vi "Main.vi"(11 "Module Admin":refnum<class "Delacor_lib_QMH_Cloneable Module Admin.lvclass">) -> ()   [LabVIEW 2020, in "TCP Client.lvlib"]
doc: "This template is based off of the Queued Message Handler design pattern and the Queued Message Handler project template that ships with LabVIEW.\n\nThe main difference is that the queue is private to this module and communication between modules is performed via Broadcast and Request events.\n\nRequest events are wrapped in public API methods and are handled in the Event Handling Loop (EHL) of this VI. Any module can register for Broadcast events sent by this module. The EHL generates messages based on user interface actions.\n\nThe Message Handling Loop (MHL) processes messages generated by the EHL, or by other messages. The messages are string values, so new messages can be added easily to the Message Cases case structure in the MHL. Each message cluster can also provide an optional value for Message Data, which is a variant that can be converted to whatever message-specific data is required.\n_____\nBased on Delacor QMH Project Template 6.0.0.89."
uses:
  TCP Client.lvlib
  <vilib>/Delacor/Delacor QMH/Libraries/Cloneable Module Admin_class/Delacor_lib_QMH_Cloneable Module Admin.lvclass
  C:/Program Files (x86)/National Instruments/LabVIEW 2020/vi.lib/Delacor/Delacor QMH/Libraries/Module Admin_class/Delacor_lib_QMH_Module Admin.lvclass
  Module Data--cluster.ctl
  <vilib>/Delacor/Delacor QMH/Libraries/Message Queue_class/Delacor_lib_QMH_Message Queue.lvclass/Delacor_lib_QMH_Message Queue.ctl
  <vilib>/Delacor/Delacor QMH/Libraries/Cloneable Module Admin_class/Delacor_lib_QMH_Cloneable Module Admin.lvclass/Delacor_lib_QMH_Cloneable Module Admin.ctl
  Stop Argument--cluster.ctl
  <vilib>/Delacor/Delacor QMH/Libraries/Module Admin_class/Delacor_lib_QMH_Module Admin.lvclass/Delacor_lib_QMH_Module Admin.ctl
  <vilib>/Utility/miscctls.llb/LVPointTypeDef.ctl
  <vilib>/Delacor/Delacor QMH/Libraries/Message Queue_class/Delacor_lib_QMH_Enqueue Message (Single).vi
  <vilib>/Delacor/Delacor QMH/Libraries/Cloneable Module Admin_class/Delacor_lib_QMH_Get Module ID.vi
  <vilib>/Delacor/Delacor QMH/Libraries/Module Admin_class/Delacor_lib_QMH_Get External Launch.vi
  <vilib>/Utility/error.llb/Error Cluster From Error Code.vi
  <vilib>/ErrorRing/Error Ring.xnode
  <vilib>/Delacor/Delacor QMH/Libraries/Message Queue_class/Delacor_lib_QMH_Message Queue.lvclass
panel:
  out "DATA":T1 {"Knob" scale=0.0..10.0; "Horizontal Pointer Slide" scale=0.0..10.0}
  in  "stop":bool
  out "error out":errorcluster
  out "Status":string
  in  "Simulate EHL Error":bool
  in  "Simulate MHL Error":bool
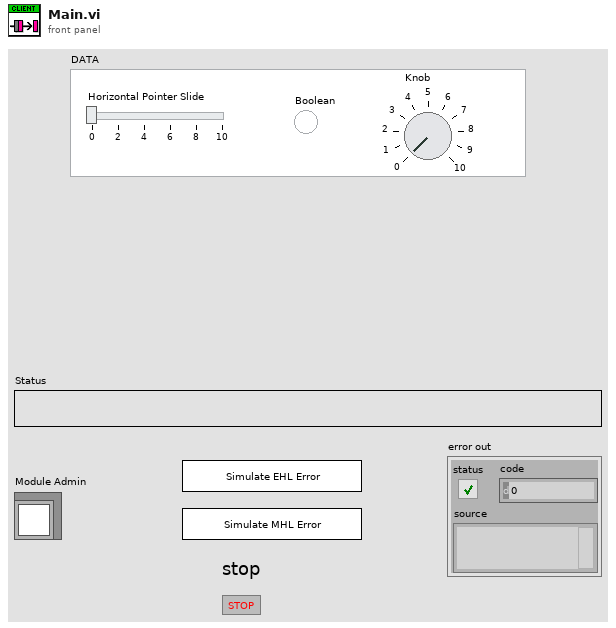
[diagram p1: front panel]
types:
  T1 = cluster{"Horizontal Pointer Slide":dbl, "Boolean":bool, "Knob":dbl}
  T2 = typedef "TCP Client.lvlib/Request Events--cluster.ctl" = cluster{"Stop Module":refnum<user-event>, "Show Panel":refnum<user-event>, "Hide Panel":refnum<user-event>, "Show Diagram":refnum<user-event>, "Get Module Execution Status":refnum<user-event>, "Connect to TCP Server":refnum<user-event>}
  T3 = typedef "TCP Client.lvlib/Module Data--cluster.ctl" = cluster{"Status":string}
  T4 = enum32{"invalid lock state", "Not Locked", "Locked (No Password)", "Password-protected"}
  T5 = typedef "TCP Client.lvlib/Stop Argument--cluster.ctl" = cluster{"Module ID":i32, "Origin":string, "Exit via Stop Module Req?":bool, "Wait for Module to stop?":bool}
  T6 = typedef "LVPointTypeDef.ctl" = cluster{"Horizontal":i16, "Vertical":i16}
  T7 = enum32{"Invalid", "Standard", "Closed", "Hidden", "Minimized", "Maximized"}
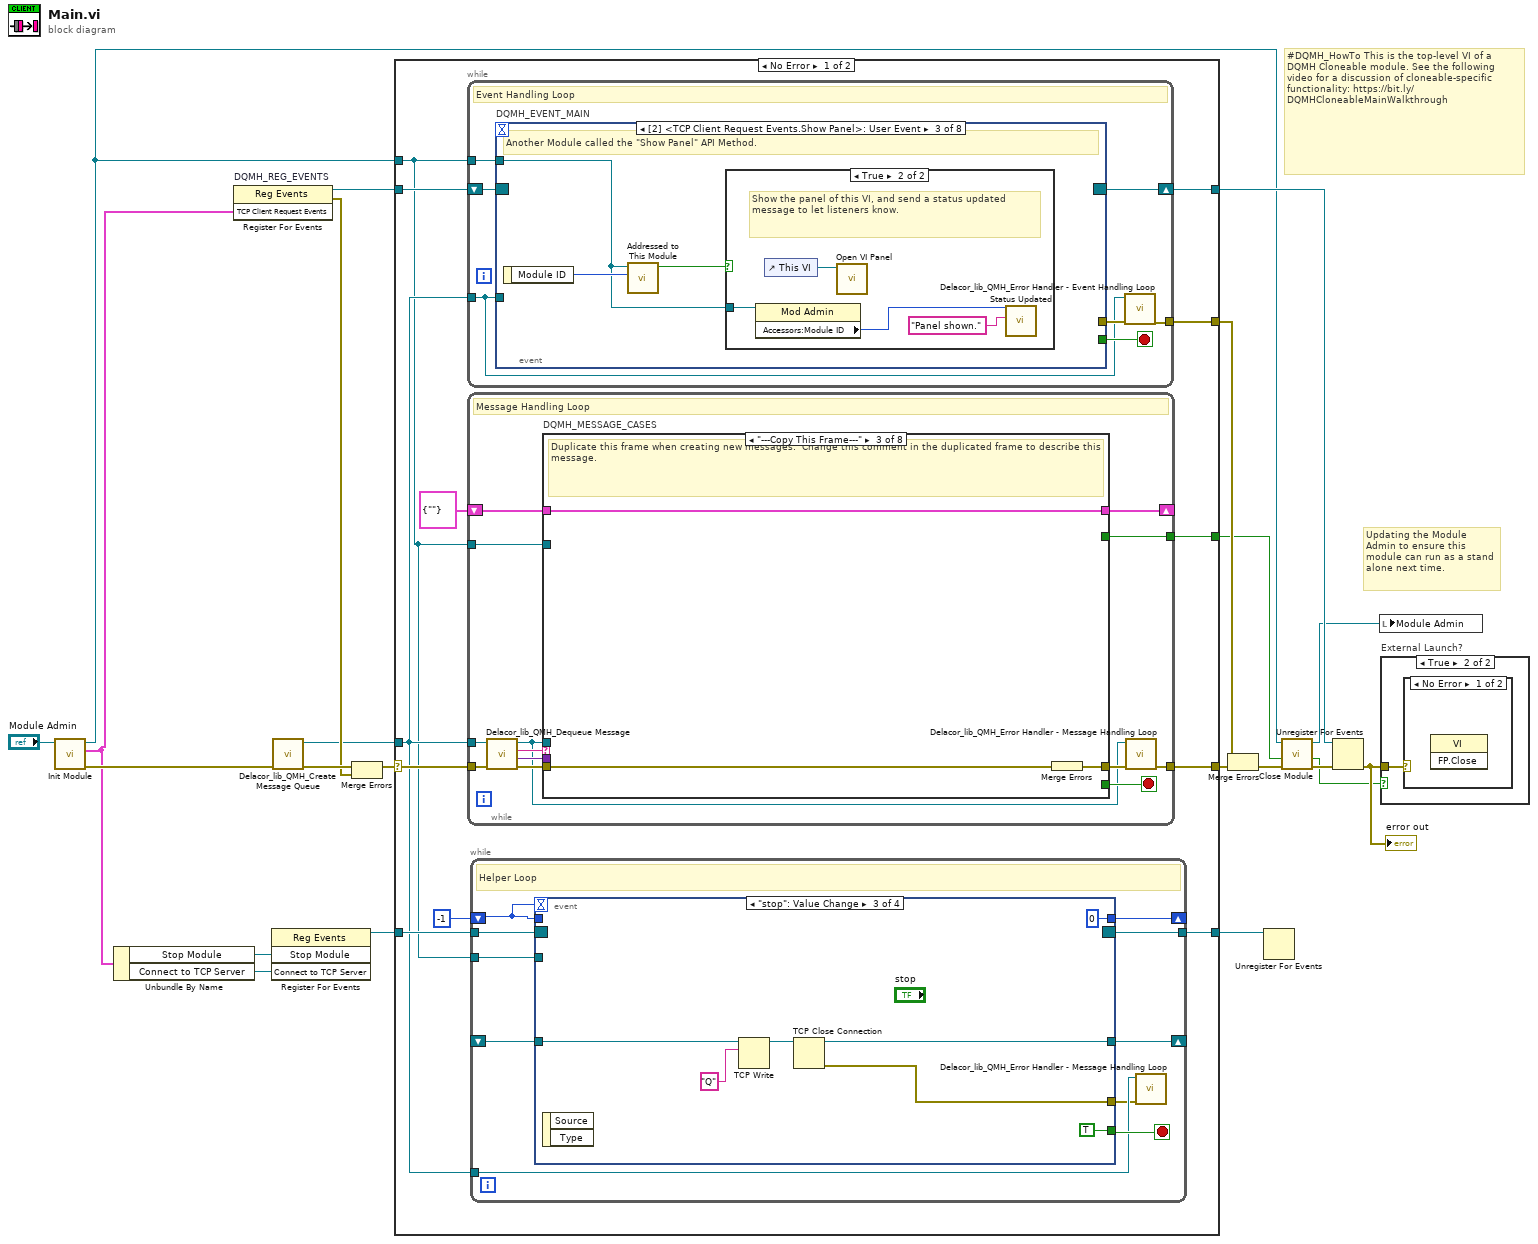
[diagram p0: block diagram]
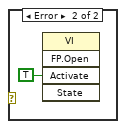
[diagram p3: hidden frame]
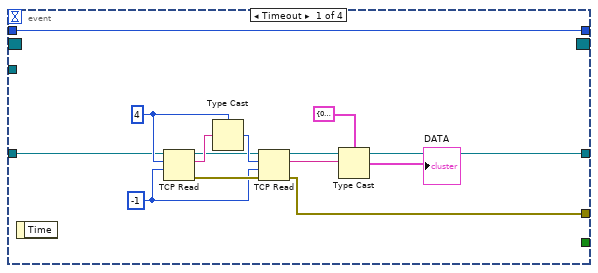
[diagram p4: hidden frame]
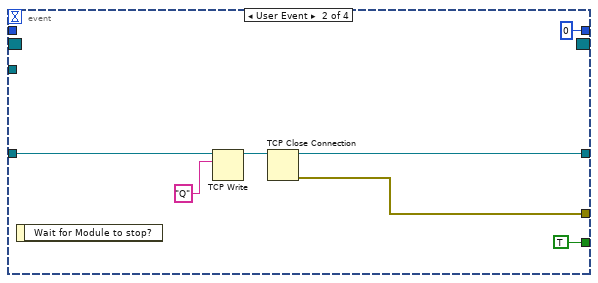
[diagram p5: hidden frame]
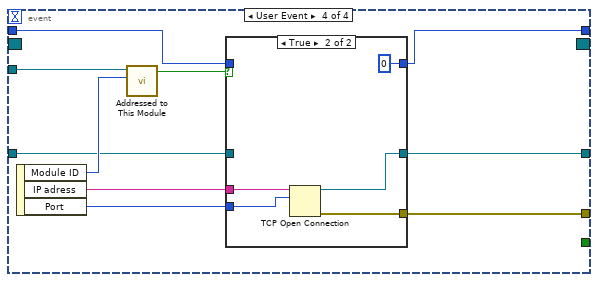
[diagram p6: hidden frame]
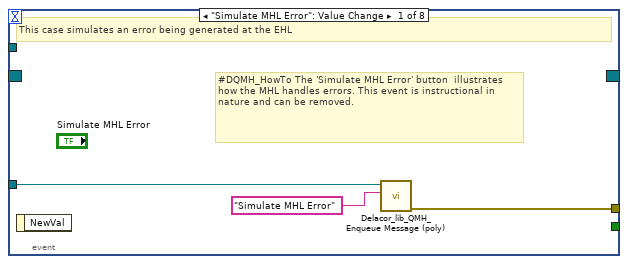
[diagram p8: hidden frame]
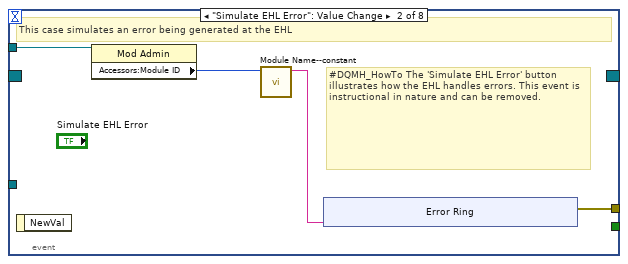
[diagram p9: hidden frame]
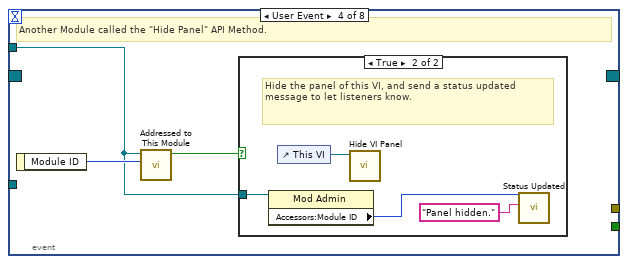
[diagram p11: hidden frame]
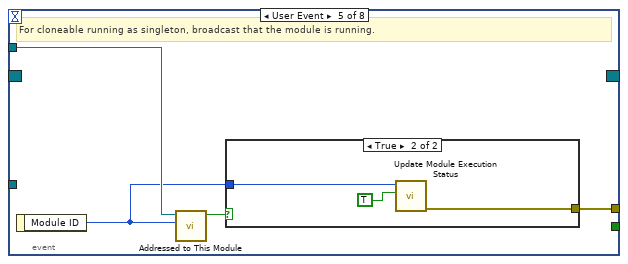
[diagram p13: hidden frame]
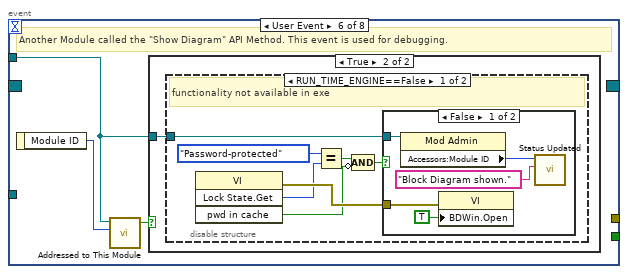
[diagram p15: hidden frame]
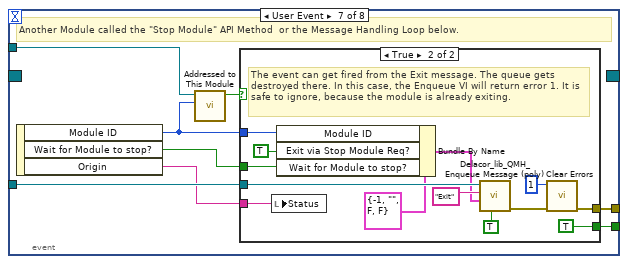
[diagram p19: hidden frame]
diagram:
  # "#DQMH_HowTo This is the top-level VI of a DQMH Cloneable module. See the following video for a discussion of cloneable-specific functionality: https://bit.ly/DQMHCloneableMainWalkthrough"
  # "Updating the Module Admin to ensure this module can run as a stand alone next time."
  n1 = call "Init Module.vi"("Cloneable Module Admin in"="Module Admin") -> ("error out"=w19:errorcluster, "TCP Client Request Events"=w5:T2, "Cloneable Module Admin out"=w9:refnum<class "Delacor_lib_QMH_Cloneable Module Admin.lvclass">)  [unwired: 8 in]
  n2 = Unbundle By Name(w5) -> ("Stop Module"=w4:refnum<user-event>, "Connect to TCP Server"=w1:refnum<user-event>)
  n3 = register-events "DQMH_REG_EVENTS"(w5) -> (reference out=w12:refnum<event-registration>, error out=w14:errorcluster)  [unwired: 2 in]
  n4 = register-events(w4, w1) -> (reference out=w3:refnum<event-registration>)  [unwired: 2 in, 1 out]
  n5 = call <vilib>:"Delacor_lib_QMH_Create Message Queue.vi"("error in"=w19) -> ("error out"=w16:errorcluster, "Message Queue"=w11:refnum<class "Delacor_lib_QMH_Message Queue.lvclass">)  [unwired: 9 in]
  n6 = Merge Errors(w16, w14) -> (w15:errorcluster)
  n7 = case shown="No Error" w15 {
    selector: w15 -> [w32 w285]
    tunnel: [w34 w284] -> w20
    tunnel: [w31 w292] -> w13
    tunnel: w12 -> [w29 w292]
    tunnel: w11 -> [w25 w283]
    tunnel: [w33 _] -> w21
    tunnel: w9 -> [w24 w288]
    tunnel: [w28 _] -> w7
    tunnel: w3 -> [w27 w282]
    tunnel: [w26 w282] -> w2
    frame No Error {
      n8 = while {
        tunnel: w25 -> [w89]
        shift-right: [w92] -> w31
        shift-left: w29 -> [w93]
        tunnel: [w94] -> w33
        tunnel: w24 -> [w90]
        stop <- w91 stop-if-true
        # "Event Handling Loop"
        n9 = event "DQMH_EVENT_MAIN" shown="[2] <TCP Client Request Events.Show Panel>: User Event" {
          selector: w93 -> [_ _ _ _ _ _ _ _]
          dyn-events: [_ _ _ _ _ _ _ _] -> w92
          timeout: _ -> [_ _ _ _ _ _ _ _]
          tunnel: [_ _ _ _ _ _ w150 _] -> w91
          tunnel: w89 -> [w97 _ _ _ _ _ w153 w169]
          tunnel: [w98 w102 _ _ w127 _ w154 w172] -> w95
          tunnel: w90 -> [_ w101 w110 w117 w125 w131 w152 w170]
          event "Simulate MHL Error": Value Change {
            # "#DQMH_HowTo The 'Simulate MHL Error' button  illustrates how the MHL handles errors. This event is instructional in nature and can be removed."
            # "This case simulates an error being generated at the EHL"
            n10 = event-data() -> ()  [unwired: 1 in, 1 out]
            n11 = call-poly <vilib>:"Delacor_lib_QMH_Enqueue Message (poly).vi"("Message"="Simulate MHL Error", "Message Queue in"=w97) -> ("error out"=w98:errorcluster)  [unwired: 8 in, 1 out]
          }
          event "Simulate EHL Error": Value Change {
            # "#DQMH_HowTo The 'Simulate EHL Error' button  illustrates how the EHL handles errors. This event is instructional in nature and can be removed."
            # "This case simulates an error being generated at the EHL"
            n12 = event-data() -> ()  [unwired: 1 in, 1 out]
            n13 = property class="Mod Admin"(reference=w101) -> ("Accessors:Module ID"=w100:i32)  [unwired: 1 in, 2 out]
            n14 = call "Module Name--constant.vi"("Module ID"=w100) -> ("Module Name"=w99:string)  [unwired: 10 in]
            n15 = xnode "Error Ring"("parameter 0"=w99) -> ("error out"=w102:errorcluster)
          }
          event User Event {
            # "Another Module called the \"Show Panel\" API Method."
            n16 = event-data() -> ("Module ID"=w111:i32)  [unwired: 1 in]
            n17 = call "Addressed to This Module.vi"("Module ID from Argument"=w111, "Module Admin"=w110) -> ("Addressed to this instance?"=w112:bool)  [unwired: 8 in, 1 out]
            n18 = case shown="True" w112 {
              tunnel: w110 -> [_ w114]
              frame False {
              }
              frame True {
                # "Show the panel of this VI, and send a status updated message to let listeners know."
                n19 = property class="Mod Admin"(reference=w114) -> ("Accessors:Module ID"=w113:i32)  [unwired: 1 in, 2 out]
                n20 = control-ref of="This VI"() -> (w116:refnum<vi>)
                n21 = call "Open VI Panel.vi"("VI"=w116) -> ()  [unwired: 10 in, 1 out]
                n22 = call "Status Updated.vi"("Status"="Panel shown." ("format string"), "Module ID"=w113) -> ()  [unwired: 9 in, 1 out]
              }
            }
          }
          event User Event {
            # "Another Module called the \"Hide Panel\" API Method."
            n23 = event-data() -> ("Module ID"=w118:i32)  [unwired: 1 in]
            n24 = call "Addressed to This Module.vi"("Module ID from Argument"=w118, "Module Admin"=w117) -> ("Addressed to this instance?"=w119:bool)  [unwired: 8 in, 1 out]
            n25 = case shown="True" w119 {
              tunnel: w117 -> [_ w121]
              frame False {
              }
              frame True {
                # "Hide the panel of this VI, and send a status updated message to let listeners know."
                n26 = property class="Mod Admin"(reference=w121) -> ("Accessors:Module ID"=w120:i32)  [unwired: 1 in, 2 out]
                n27 = control-ref of="This VI"() -> (w123:refnum<vi>)
                n28 = call "Hide VI Panel.vi"("VI"=w123) -> ()  [unwired: 10 in, 1 out]
                n29 = call "Status Updated.vi"("Status"="Panel hidden." ("format string"), "Module ID"=w120) -> ()  [unwired: 9 in, 1 out]
              }
            }
          }
          event User Event {
            # "For cloneable running as singleton, broadcast that the module is running."
            n30 = event-data() -> ("Module ID"=w124:i32)  [unwired: 1 in]
            n31 = call "Addressed to This Module.vi"("Module ID from Argument"=w124, "Module Admin"=w125) -> ("Addressed to this instance?"=w126:bool)  [unwired: 8 in, 1 out]
            n32 = case shown="True" w126 {
              tunnel: [_ w130] -> w127
              tunnel: w124 -> [_ w129]
              frame False {
              }
              frame True {
                n33 = call "Update Module Execution Status.vi"("Running?"=TRUE, "Module ID"=w129) -> ("error out"=w130:errorcluster)  [unwired: 9 in]
              }
            }
          }
          event User Event {
            # "Another Module called the \"Show Diagram\" API Method. This event is used for debugging."
            n34 = event-data() -> ("Module ID"=w132:i32)  [unwired: 1 in]
            n35 = call "Addressed to This Module.vi"("Module ID from Argument"=w132, "Module Admin"=w131) -> ("Addressed to this instance?"=w133:bool)  [unwired: 8 in, 1 out]
            n36 = case shown="True" w133 {
              tunnel: w131 -> [_ w134]
              frame False {
              }
              frame True {
                n37 = disable-structure shown="RUN_TIME_ENGINE==False" {
                  disable-tunnel: w134 -> [w135 _]
                  frame condition #0 (active) {
                    # "functionality not available in exe"
                    n38 = invoke class="VI" method="Lock State.Get"() -> (error out=w141:errorcluster, "Get Lock State"=w140:T4, "pwd in cache"=w137:bool)  [unwired: 4 in, 1 out]
                    n39 = Equal?(x=T4."Password-protected", y=w140) -> (x = y?=w138:bool)
                    n40 = Compound Arithmetic op=AND(w138, invert w137) -> (w136:bool)
                    n41 = case shown="False" w136 {
                      tunnel: w141 -> [w146 _]
                      tunnel: w135 -> [w143 _]
                      frame False {
                        n42 = property class="Mod Admin"(reference=w143) -> ("Accessors:Module ID"=w142:i32)  [unwired: 1 in, 2 out]
                        n43 = property class="VI"(error in=w146, "BDWin.Open"=TRUE ("Block Diagram Window:Open")) -> ()  [unwired: 1 in, 2 out]
                        n44 = call "Status Updated.vi"("Status"="Block Diagram shown." ("format string"), "Module ID"=w142) -> ()  [unwired: 9 in, 1 out]
                      }
                      frame True {
                        # "Password-protected VI, and the password is not in the cache. Do not show the diagram."
                      }
                    }
                  }
                  frame condition #1 {
                  }
                }
              }
            }
          }
          event User Event {
            # "Another Module called the \"Stop Module\" API Method  or the Message Handling Loop below."
            n45 = event-data() -> ("Module ID"=w148:i32, "Wait for Module to stop?"=w149:bool, "Origin"=w147:string)  [unwired: 1 in]
            n46 = call "Addressed to This Module.vi"("Module ID from Argument"=w148, "Module Admin"=w152) -> ("Addressed to this instance?"=w151:bool)  [unwired: 8 in, 1 out]
            n47 = case shown="True" w151 {
              tunnel: [_ w166] -> w154
              tunnel: w153 -> [_ w162]
              tunnel: [_ TRUE] -> w150
              tunnel: w149 -> [_ w157]
              tunnel: w148 -> [_ w159]
              tunnel: w147 -> [_ w155]
              frame False {
              }
              frame True {
                # "The event can get fired from the Exit message. The queue gets destroyed there. In this case, the Enqueue VI will return error 1. It is safe to ignore, because the module is already exiting."
                n48 = local write "Status"(w155) -> ()
                n49 = Bundle By Name(cluster=T5 {"Module ID"=-1, "Origin"="", "Exit via Stop Module Req?"=FALSE, "Wait for Module to stop?"=FALSE} ("Stop Argument"), "Module ID"=w159, "Exit via Stop Module Req?"=TRUE, "Wait for Module to stop?"=w157) -> (w156:T5)
                n50 = call-poly <vilib>:"Delacor_lib_QMH_Enqueue Message (poly).vi"("Priority Message? (F)"=TRUE, "Message Data"=w156, "Message"="Exit", "Message Queue in"=w162) -> ("error out"=w167:errorcluster)  [unwired: 6 in, 1 out]
                n51 = call <vilib>:"Clear Errors.vi"("error in (no error)"=w167, "specific error code to clear (0: all)"=1) -> ("error out"=w166:errorcluster)  [unwired: 4 in, 1 out]
              }
            }
          }
          event Panel Close? {
            w171 = TRUE  # Discard the event, the MHL is responsible for closing and stopping this VI.
            # "Hide the panel or send the 'Exit' message if the user clicks the 'X' on the module main VI panel."
            n52 = event-data() -> ()  [unwired: 1 in, 1 out]
            n53 = property class="Mod Admin"(reference=w170) -> ("Accessors:External Launch"=w168:bool)  [unwired: 1 in, 2 out]
            n54 = case shown="True" w168 {
              tunnel: w169 -> [_ w176]
              tunnel: [_ w177] -> w172
              frame True {
                # "If externally launched, clicking the 'X' hides the panel, but doesn't close it."
                n55 = control-ref of="This VI"() -> (w173:refnum<vi>)
                n56 = call "Hide VI Panel.vi"("VI"=w173) -> ()  [unwired: 10 in, 1 out]
              }
              frame False {
                # "If run as a stand-alone VI, clicking the panel 'X' stops the VI."
                n57 = call-poly <vilib>:"Delacor_lib_QMH_Enqueue Message (poly).vi"("Priority Message? (F)"=TRUE, "Message"="Exit", "Message Queue in"=w176) -> ("error out"=w177:errorcluster)  [unwired: 7 in, 1 out]
              }
            }
            n58 = event-data("Discard?"=w171) -> ()  [unwired: 1 in, 1 out]
          }
        }
        n59 = call-dynamic "Delacor_lib_QMH_Error Handler - Event Handling Loop.vi"("error in"=w95, "Message Queue in"=w89) -> ("dup error in"=w94:errorcluster)  [unwired: 8 in, 1 out]
      }
      n60 = while {
        tunnel: w25 -> [w181]
        shift-right: [w185] -> _
        shift-left: T3 {"Status"=""} ("Data Cluster") -> [w186]
        tunnel: w32 -> [w189]
        tunnel: [w187] -> w34
        tunnel: w24 -> [w179]
        tunnel: [w178] -> w28
        stop <- w184 stop-if-true
        # "Message Handling Loop"
        n61 = call-dynamic "Delacor_lib_QMH_Dequeue Message.vi"("error in"=w189, "Message Queue in"=w181) -> ("error out"=w188:errorcluster, "Message Data"=w182:variant, "Message"=w183:string, "Message Queue out"=w180:refnum<class "Delacor_lib_QMH_Message Queue.lvclass">)  [unwired: 6 in]
        n62 = case "DQMH_MESSAGE_CASES" shown="\"---Copy This Frame---\"" w183 {
          selector: w183 -> [_ _ _ _ _ _ _ w269]
          tunnel: w180 -> [_ _ _ _ w220 _ w259 _]
          tunnel: w188 -> [w209 w213 w216 w218 w229 w242 w265 w271]
          tunnel: [w207 w213 w215 w218 w225 w241 w262 w272] -> w190
          tunnel: w186 -> [w200 w212 w214 w217 w224 w239 w258 w270]
          tunnel: [w199 w212 w214 w217 w224 w239 w258 w270] -> w185
          tunnel: [_ _ _ _ _ _ w257 _] -> w184
          tunnel: w182 -> [_ _ _ _ w223 _ w255 _]
          tunnel: w179 -> [w194 _ _ _ w222 w237 w251 w267]
          tunnel: [_ _ _ _ _ _ w253 _] -> w178
          frame "Initialize" {
            w191 = "Initial Message" ("Initial Message")
            # "#CodeNeeded - Initialize the appearance of the front panel."
            # "#CodeNeeded - Initialize your state data here."
            # "Initialize - Any operation that needs to be done before the module can receive messages. Synchronize Caller Events.vi will inform Start Module.vi that the module has launched and is ready to receive messages. Module Did Init.vi will broadcast that the module initialized."
            n63 = call "Synchronize Caller Events.vi"("error in (no error)"=w209, "Module Admin"=w194) -> ("error out"=w208:errorcluster, "Module Admin out"=w193:refnum<class "Delacor_lib_QMH_Cloneable Module Admin.lvclass">)  [unwired: 8 in]
            n64 = property class="Mod Admin"(reference=w193) -> ("Accessors:Module ID"=w196:i32, "Accessors:External Launch"=w195:bool)  [unwired: 1 in, 2 out]
            n65 = call "Module Name--constant.vi"("Module ID"=w196) -> ("Module Name"=w204:string)  [unwired: 10 in]
            n66 = property class="VI"("Front Panel.Title"=w204) -> (reference out=w206:refnum<vi>, error out=w211:errorcluster)  [unwired: 2 in]
            n67 = Select(t=T7."Hidden" ("State"), s=w195, f=T7."Standard" ("State")) -> (s? t:f=w201:T7)
            n68 = invoke class="VI" method="FP.Open"(reference=w206, error in=w211, "State"=w201) -> (reference out=w205:refnum<vi>, error out=w210:errorcluster)  [unwired: 2 in, 3 out]
            n69 = call "Module Name--constant.vi"("Module ID"=w196) -> ("Module Name"=w197:string)  [unwired: 10 in]
            n70 = Bundle By Name(cluster=w200, "Status"=w191) -> (w199:T3)
            n71 = invoke class="VI" method="FP.Center"(reference=w205, error in=w210) -> ()  [unwired: 1 in, 3 out]
            n72 = property on="Pane" class="Pane"("Origin"=T6 {"Horizontal"=0, "Vertical"=0}) -> ()  [unwired: 2 in, 2 out]
            n73 = call "Module Did Init.vi"("error in (no error)"=w208, "Initialized?"=TRUE, "Origin"=w197, "Module ID"=w196) -> ("error out"=w207:errorcluster)  [unwired: 7 in]
            "Status" <- w191
          }
          frame "---Module Specific---" {
            # "Separator -- The following cases handle messages specific to this Module."
          }
          frame "---Copy This Frame---" {
            # "Duplicate this frame when creating new messages.  Change this comment in the duplicated frame to describe this message."
            n74 = Merge Errors(w216) -> (w215:errorcluster)
          }
          frame "---Exit and Error Handling---" {
            # "Separator - the following cases handle errors and exit messages."
          }
          frame "Error" {
            # "#CodeRecommended - If you ever change the name of this \"Error\" message, you'll need to update the name in the Check Loop Error.vi as well."
            # "#CodeRecommended - If the module is running in standalone mode (External Launch = FALSE), this code will pop up an error dialog and call the 'Exit' message if an error occurs. Add more fine-grained error handling here."
            # "Error - Check the error message data and respond accordingly. This message is sent by the \"Error Handler\" VIs at the end of each loop in this application."
            n75 = property class="Mod Admin"(reference=w222) -> ("Accessors:External Launch"=w221:bool, "Accessors:Module ID"=w219:i32)  [unwired: 1 in, 2 out]
            n76 = Variant To Data(error in=w229, type=errorcluster {"status"=FALSE, "code"=0, "source"=""} ("error constant"), Variant=w223) -> (data=w230:errorcluster, error out=w227:errorcluster)
            n77 = call "Error Reported.vi"("Error"=w230, "Module ID"=w219) -> ()  [unwired: 9 in, 1 out]
            n78 = case shown="False" w221 {
              tunnel: [w235 _] -> w226
              tunnel: w220 -> [w233 _]
              tunnel: w230 -> [w234 _]
              frame False {
                # "If the module is running standalone, then pop up an error dialog and call the \"Exit\" message."
                n79 = call <vilib>:"Simple Error Handler.vi"("error in (no error)"=w234) -> ()  [unwired: 4 in, 5 out]
                n80 = call-poly <vilib>:"Delacor_lib_QMH_Enqueue Message (poly).vi"("Priority Message? (F)"=TRUE, "Message"="Exit", "Message Queue in"=w233) -> ("error out"=w235:errorcluster)  [unwired: 7 in, 1 out]
              }
              frame True {
                # "If the module was launched externally, calling the Error Reported broadcast VI is the only action performed by the \"Error\" message. The module's caller can then process the error appropriately."
              }
            }
            n81 = Merge Errors(w227, w226) -> (w225:errorcluster)
            n82 = local write "error out"(w225) -> ()
          }
          frame "Simulate MHL Error" {
            # "#DQMH_HowTo The 'Simulate MHL Error' button  illustrates how the MHL handles errors. This event is instructional in nature and can be removed."
            # "Simulate an error occurring at the MHL"
            n83 = property class="Mod Admin"(reference=w237) -> ("Accessors:Module ID"=w238:i32)  [unwired: 1 in, 2 out]
            n84 = call "Module Name--constant.vi"("Module ID"=w238) -> ("Module Name"=w236:string)  [unwired: 10 in]
            n85 = xnode "Error Ring"("parameter 0"=w236) -> ("error out"=w240:errorcluster)
            n86 = Merge Errors(w242, w240) -> (w241:errorcluster)
          }
          frame "Exit" {
            w256 = 91  # 91: not all Exit messages will have an argument
            w257 = TRUE  # Stop the VI
            # "Release the message queue reference"
            # "#CodeNeeded - Add any required cleanup code here."
            # "Exit - Exit the application."
            n87 = Variant To Data(error in=w265, type=T5 {"Module ID"=-1, "Origin"="", "Exit via Stop Module Req?"=FALSE, "Wait for Module to stop?"=FALSE} ("Stop Argument"), Variant=w255) -> (data=w252:T5, error out=w260:errorcluster)
            n88 = call <vilib>:"Clear Errors.vi"("error in (no error)"=w260, "specific error code to clear (0: all)"=w256) -> ("error out"=w264:errorcluster)  [unwired: 4 in, 1 out]
            n89 = control-ref of="This VI"() -> (w250:refnum<vi>)
            n90 = call-dynamic "Delacor_lib_QMH_Release Message Queue.vi"("error in"=w264, "Message Queue"=w259) -> ("error out"=w263:errorcluster)  [unwired: 9 in]
            n91 = call "Handle Exit.vi"("Stop Argument"=w252, "Module Admin in"=w251, "VI reference"=w250) -> ("error out"=w261:errorcluster, "Wait for Stop?"=w253:bool)  [unwired: 7 in]
            n92 = Merge Errors(w263, w261) -> (w262:errorcluster)
          }
          frame Default {
            # "'Default' case only runs if there is a message that isn't defined in any of the other cases.  Output a programming error."
            n93 = property class="Mod Admin"(reference=w267) -> ("Accessors:Module ID"=w266:i32)  [unwired: 1 in, 2 out]
            n94 = call "Module Name--constant.vi"("Module ID"=w266) -> ("Module Name"=w268:string)  [unwired: 10 in]
            n95 = xnode "Error Ring"("parameter 0"=w269, "parameter 1"=w268) -> ("error out"=w273:errorcluster)
            n96 = Merge Errors(w271, w273) -> (w272:errorcluster)
          }
        }
        n97 = call-dynamic "Delacor_lib_QMH_Error Handler - Message Handling Loop.vi"("error in"=w190, "Message Queue in"=w180) -> ("dup error in"=w187:errorcluster)  [unwired: 8 in, 1 out]
      }
      n98 = while {
        tunnel: w27 -> [w44]
        tunnel: [w42] -> w26
        tunnel: w25 -> [w41]
        tunnel: w24 -> [w40]
        shift-right: [w38] -> _
        shift-left: _ -> [w37]
        shift-right: [w35] -> _
        shift-left: -1 -> [w36]
        stop <- w43 stop-if-true
        # "Helper Loop"
        n99 = event shown="[2] \"stop\": Value Change" {
          selector: w44 -> [_ _ _ _]
          dyn-events: [_ _ _ _] -> w42
          timeout: w36 -> [_ _ _ _]
          tunnel: [_ TRUE TRUE _] -> w43
          tunnel: w40 -> [_ _ _ w78]
          tunnel: [w50 w62 w69 w76] -> w39
          tunnel: [w48 w63 w70 w75] -> w38
          tunnel: w37 -> [w49 w60 w67 w74]
          tunnel: w36 -> [w57 _ _ w73]
          tunnel: [w57 0 0 w72] -> w35
          event Timeout {
            w51 = -1
            w52 = 4
            n100 = event-data() -> ()  [unwired: 1 in, 1 out]
            n101 = TCP Read(connection ID=w49, bytes to read=w52, 9:w51) -> (connection ID out=w53:refnum<k5>, data out=w56:string, error out=w55:errorcluster)  [unwired: 1 in, 1 out]
            n102 = Type Cast(type=w52, x=w56) -> (*(type *) &x=w54:i32)
            n103 = TCP Read(connection ID=w53, bytes to read=w54, error in (no error)=w55, 9:w51) -> (connection ID out=w48:refnum<k5>, data out=w47:string, error out=w50:errorcluster)  [unwired: 1 out]
            n104 = Type Cast(type=T1 {"Horizontal Pointer Slide"=0.0, "Boolean"=FALSE, "Knob"=0.0} ("DATA"), x=w47) -> (*(type *) &x=→"DATA":T1)
          }
          event User Event {
            n105 = event-data() -> ()  [unwired: 1 in, 1 out]
            n106 = TCP Write(connection ID=w60, data in="Q") -> (connection ID out=w59:refnum<k5>)  [unwired: 1 in, 3 out]
            n107 = TCP Close Connection(connection ID=w59) -> (connection ID out=w63:refnum<k5>, error out=w62:errorcluster)  [unwired: 1 in, 1 out]
          }
          event "stop": Value Change {
            n108 = event-data() -> ()  [unwired: 1 in, 2 out]
            n109 = TCP Write(connection ID=w67, data in="Q") -> (connection ID out=w66:refnum<k5>)  [unwired: 1 in, 3 out]
            n110 = TCP Close Connection(connection ID=w66) -> (connection ID out=w70:refnum<k5>, error out=w69:errorcluster)  [unwired: 1 in, 1 out]
          }
          event User Event {
            n111 = event-data() -> ("Module ID"=w79:i32, "IP adress"=w81:string, "Port"=w80:u16)  [unwired: 1 in]
            n112 = call "Addressed to This Module.vi"("Module ID from Argument"=w79, "Module Admin"=w78) -> ("Addressed to this instance?"=w77:bool)  [unwired: 8 in, 1 out]
            n113 = case shown="True" w77 {
              tunnel: w81 -> [_ w88]
              tunnel: w80 -> [_ w87]
              tunnel: [_ w86] -> w76
              tunnel: [w83 w85] -> w75
              tunnel: w74 -> [w83 _]
              tunnel: w73 -> [w82 _]
              tunnel: [w82 0] -> w72
              frame False {
              }
              frame True {
                n114 = TCP Open Connection(address=w88, remote port or service name=w87) -> (connection ID=w85:refnum<k5>, error out=w86:errorcluster)  [unwired: 1 in, 2 out]
              }
            }
          }
        }
        n115 = call-dynamic "Delacor_lib_QMH_Error Handler - Message Handling Loop.vi"("error in"=w39, "Message Queue in"=w41) -> ()  [unwired: 8 in, 2 out]
      }
    }
    frame Error {
      n116 = call "Synchronize Caller Events.vi"("Module Admin"=w288) -> ("Module Admin out"=w287:refnum<class "Delacor_lib_QMH_Cloneable Module Admin.lvclass">)  [unwired: 9 in, 1 out]
      n117 = property class="Mod Admin"(reference=w287) -> ("Accessors:Module ID"=w286:i32)  [unwired: 1 in, 2 out]
      n118 = call-dynamic "Delacor_lib_QMH_Release Message Queue.vi"("error in"=w285, "Message Queue"=w283) -> ("error out"=w284:errorcluster)  [unwired: 9 in]
      n119 = call "Module Name--constant.vi"("Module ID"=w286) -> ("Module Name"=w291:string)  [unwired: 10 in]
      n120 = Format Into String(format string="An error occurred during initialization. %s is no longer running.", w291) -> (resulting string=w289:string)  [unwired: 2 in, 1 out]
      n121 = call "Error Reported.vi"("Additional Information"=w289, "Error"=w284, "Module ID"=w286) -> ()  [unwired: 8 in, 1 out]
    }
  }
  n122 = Merge Errors(w21, w20) -> (w22:errorcluster)
  n123 = Unregister For Events(event registration refnum=w2) -> ()  [unwired: 1 in, 1 out]
  n124 = call "Close Module.vi"("error in"=w22, "Wait for stop?"=w7, "Module Admin in"=w9) -> ("error out"=w18:errorcluster, "External Launch"=w6:bool, "Module Admin out"=w8:refnum<class "Delacor_lib_QMH_Cloneable Module Admin.lvclass">)  [unwired: 6 in]
  n125 = Unregister For Events(event registration refnum=w13, error in=w18) -> (error out=w17:errorcluster)
  "error out" <- w17
  n126 = local write "Module Admin"(w8) -> ()
  n127 = case "External Launch?" shown="True" w6 {
    tunnel: w17 -> [_ w293]
    frame False {
    }
    frame True {
      n128 = case shown="No Error" w293 {
        frame No Error {
          n129 = invoke class="VI" method="FP.Close"() -> ()  [unwired: 3 in, 3 out]
        }
        frame Error {
          n130 = invoke class="VI" method="FP.Open"("Activate"=TRUE ("Activate?")) -> ()  [unwired: 4 in, 5 out]
        }
      }
    }
  }
